vi "ErrorDaemon.set.vi"(10 "ErrorDaemon":refnum<class "ErrorDaemon.lvclass">, 11 "TemplateDaemon in":refnum<class "TemplateDaemon.lvclass">) -> (3 "TemplateDaemon out":refnum<class "TemplateDaemon.lvclass">)   [LabVIEW 2020, in "TemplateDaemon.lvclass"]
uses:
  TemplateDaemon.lvclass
  ErrorDaemon_class/ErrorDaemon.lvclass
  TemplateDaemon.lvclass/TemplateDaemon.ctl
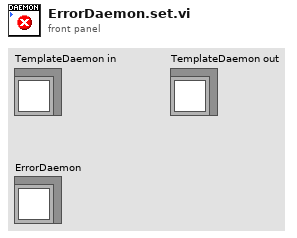
[diagram p1: front panel]
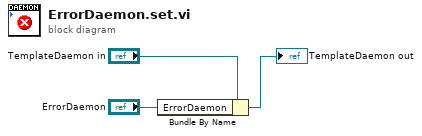
[diagram p0: block diagram]
diagram:
  n1 = Bundle By Name(cluster="TemplateDaemon in", "ErrorDaemon"="ErrorDaemon") -> (→"TemplateDaemon out":refnum<class "TemplateDaemon.lvclass">)
